vi "Scan Setup.vi"(8 "error in (no error)":errorcluster, 11 "anritsu reader in":refnum<class "anritsu reader.lvclass">) -> (0 "error out":errorcluster, 3 "anritsu reader out":refnum<class "anritsu reader.lvclass">)   [LabVIEW 2017, in "anritsu reader.lvclass"]
doc: "(Dynamic) Send commands to configure the instrument based on the class member fields."
uses:
  anritsu reader.lvclass
  Reader/Reader.lvclass
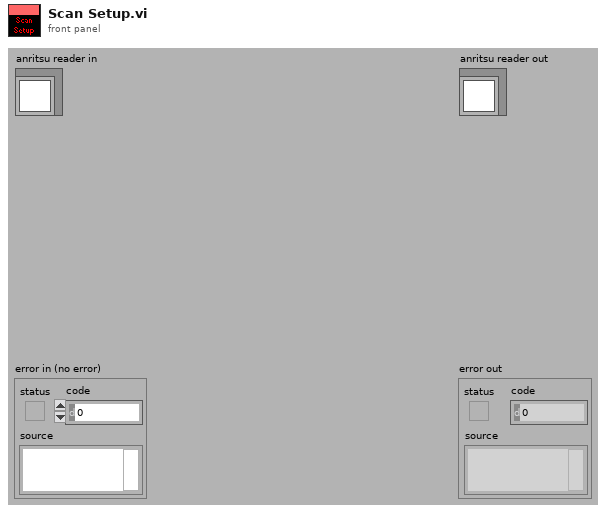
[diagram p1: front panel]
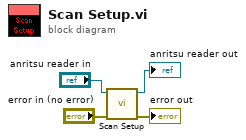
[diagram p0: block diagram]
diagram:
  n1 = call-parent "Scan Setup.vi"("error in (no error)"="error in (no error)", "Reader in"="anritsu reader in") -> ("error out"=→"error out":errorcluster, "Reader out"=→"anritsu reader out":refnum<class "anritsu reader.lvclass">)  [unwired: 8 in]
